vi "test_formatNumericToString_formatDoubleToStringUsingBigEndian.vi"(8 "error in (no error)":errorcluster, 11 "TestCase in":refnum<class "Instrument Addon Unit Test.lvclass">) -> (0 "error out":errorcluster, 3 "TestCase out":refnum<class "Instrument Addon Unit Test.lvclass">)   [LabVIEW 2019, in "Instrument Addon Unit Test.lvclass"]
uses:
  Instrument Addon Unit Test.lvclass
  Addon/Addon Shared/Types/Endian.ctl
  <vilib>/addons/_JKI Toolkits/VI Tester/TestCase.llb/TestCase.lvclass
  Addon/Addon Shared/Instrument Addon Shared.lvlib
  C:/Program Files (x86)/National Instruments/LabVIEW 2019/vi.lib/addons/_JKI Toolkits/VI Tester/TestCase.llb/TestCase.lvclass
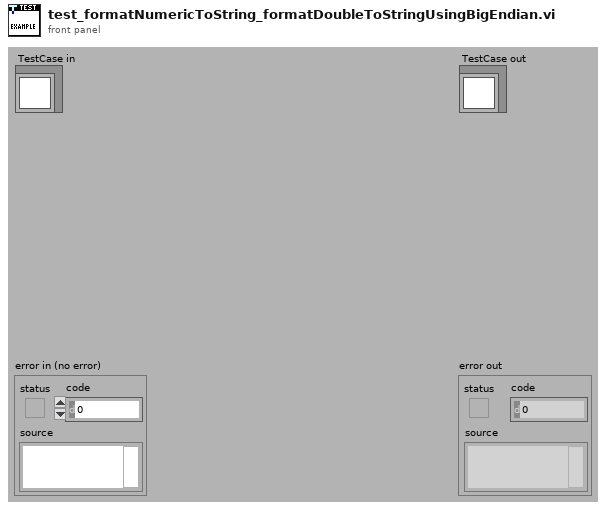
[diagram p1: front panel]
types:
  T1 = typedef "Instrument Addon Shared.lvlib/Endian.ctl" = enum16{"Native", "Little", "Big"}
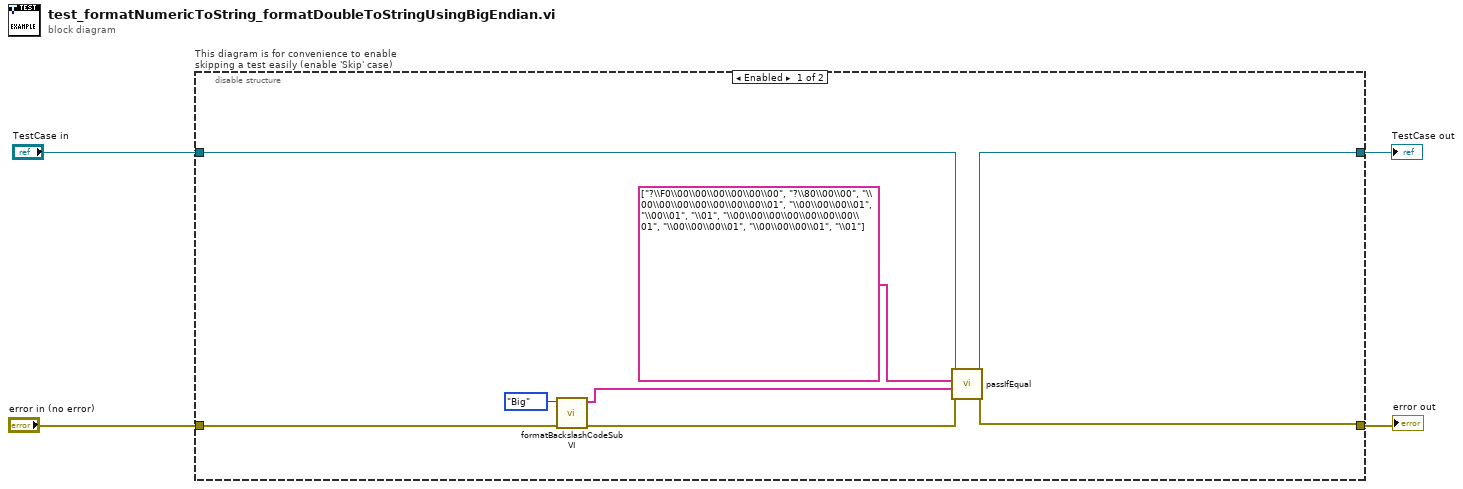
[diagram p0: block diagram]
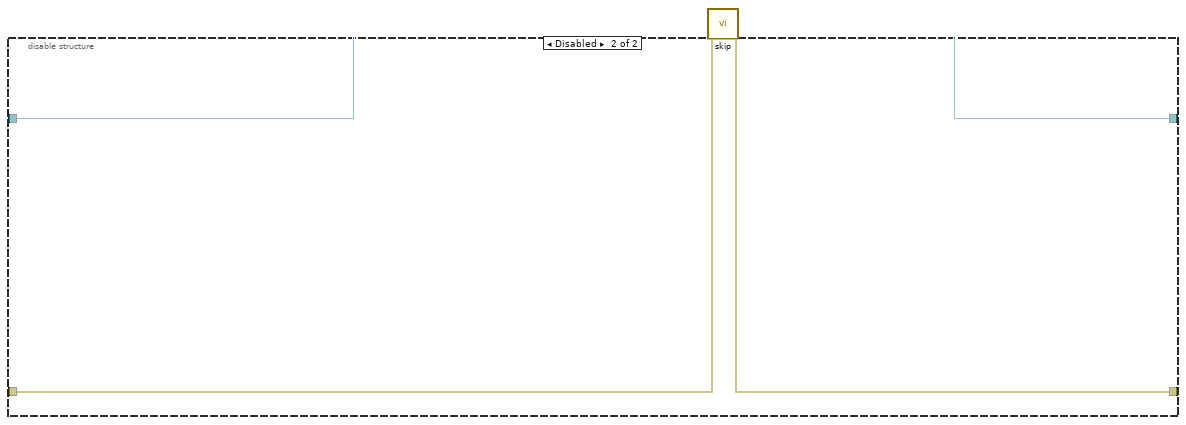
[diagram p2: hidden frame]
diagram:
  n1 = disable-structure "This diagram is for convenience to enable skipping a test easily (enable 'Skip' case)" shown="Enabled" {
    disable-tunnel: "TestCase in" -> [w12 w16]
    disable-tunnel: [w11 w14] -> w1
    disable-tunnel: [w10 w15] -> w3
    disable-tunnel: "error in (no error)" -> [w6 w13]
    frame Enabled {
      n2 = call "formatBackslashCodeSubVI.vi"("error in (no error)"=w6, "Endian"=Endian."Big") -> ("error out"=w7:errorcluster, "Values"=w8:string[])  [unwired: 8 in]
      n3 = call-dynamic "passIfEqual.vi"("error in (no error)"=w7, "y"=w8, "x"=string[] ["?\\F0\\00\\00\\00\\00\\00\\00", "?\\80\\00\\00", "\\00\\00\\00\\00\\00\\00\\00\\01", "\\00\\00\\00\\01", "\\00\\01", "\\01", "\\00\\00\\00\\00\\00\\00\\00\\01", "\\00\\00\\00\\01", "\\00\\00\\00\\01", "\\01"] ("Values"), "TestCase in"=w12) -> ("error out"=w10:errorcluster, "TestCase out"=w11:refnum<class "Instrument Addon Unit Test.lvclass">)  [unwired: 6 in]
    }
    frame Disabled {
      # "skip test result while test is under development"
      n4 = call <vilib>:"skip.vi"("error in (no error)"=w13, "TestCase in"=w16) -> ("error out"=w15:errorcluster, "TestCase out"=w14:refnum<class "Instrument Addon Unit Test.lvclass">)  [unwired: 8 in]
    }
  }
  "error out" <- w3
  "TestCase out" <- w1
